vi "SVT UFF58 Write Record 8.vi"(0 "function refnum":refnum<k20>, 5 "abscissa data characteristics":T1 {"specific data type" items=["unknown"=0, "general"=1, "stress"=2, "strain"=3, "temperature"=5, "heat flux"=6, "displacement"=8, "reaction force"=9, "velocity"=11, "acceleration"=12, "excitation force"=13, "pressure"=15, "mass"=16, "time"=17, "frequency"=18, "rpm"=19, "order"=20, "sound pressure"=21, "sound intensity"=22, "sound power"=23]}, 11 "error in (no error)":errorcluster) -> (4 "dup function refnum":refnum<k20>, 15 "error out":errorcluster)   [LabVIEW 2017, in "SoundVib_UFF58.lvlib"]
doc: "Writes the values of the fields in record 8 of the UFF58 (universal file format) file. Record 8 contains the abscissa data characteristics."
uses:
  <vilib>/addons/Sound and Vibration/svt_UFF58/SoundVib_UFF58.lvlib
  <vilib>/addons/Sound and Vibration/svt_UFF58/subVIs/sv_UFF58 Axis Characteristics.ctl
  <vilib>/addons/Sound and Vibration/svt_UFF58/subVIs/sv_UFF58 Specific Datatype.ctl
  <vilib>/Platform/storage/Storage.llb/Set Property (String).vi
  <vilib>/Platform/storage/Storage.llb/Set Property (I32).vi
  <vilib>/Platform/storage/Storage.llb/Get Property (Storage Refnums).vi
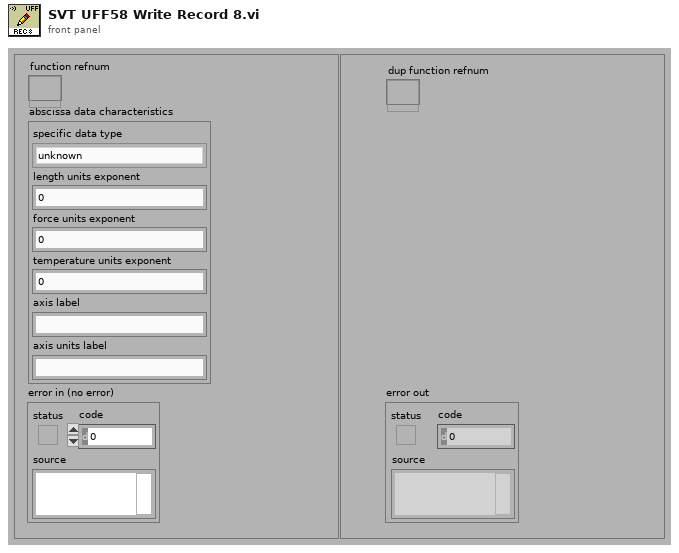
[diagram p1: front panel]
types:
  T1 = typedef "SoundVib_UFF58.lvlib/sv_UFF58 Axis Characteristics.ctl" = cluster{"specific data type":T2, "length units exponent":i32, "force units exponent":i32, "temperature units exponent":i32, "axis label":string, "axis units label":string}
  T2 = typedef "SoundVib_UFF58.lvlib/sv_UFF58 Specific Datatype.ctl" = u16
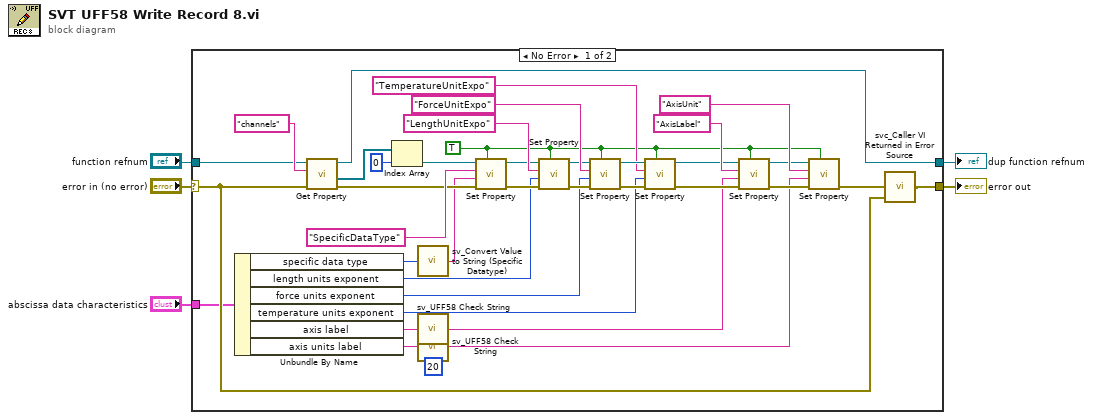
[diagram p0: block diagram]
diagram:
  n1 = case shown="No Error" "error in (no error)" {
    selector: "error in (no error)" -> [w10 w44]
    tunnel: [w12 w44] -> w5
    tunnel: "abscissa data characteristics" -> [w9 _]
    tunnel: "function refnum" -> [w17 w45]
    tunnel: [w14 w45] -> w1
    frame No Error {
      w8 = TRUE ("Create if not found (no:F)")
      w13 = 20 ("length (rest)")
      n2 = Unbundle By Name(w9) -> ("specific data type"=w6:T2, "length units exponent"=w25:i32, "force units exponent"=w24:i32, "temperature units exponent"=w23:i32, "axis label"=w27:string, "axis units label"=w26:string)
      n3 = call-poly <vilib>:"Get Property.vi"("error in (no error)"=w10, "Property name"="channels", "storage refnum"=w17) -> ("error out"=w16:errorcluster, "Value"=w19:refnum<k20>[], "storage refnum out"=w14:refnum<k20>)  [unwired: 6 in]
      n4 = Index Array(array=w19, index=0) -> (element=w15:refnum<k20>)
      n5 = call <vilib>:"sv_Convert Value to String (Specific Datatype).vi"("specific data type value"=w6) -> ("specific data type string"=w7:string)  [unwired: 14 in]
      n6 = call <vilib>:"sv_UFF58 Check String.vi"("field value"=w27, "field length"=w13) -> ("output string"=w21:string)  [unwired: 12 in, 1 out]
      n7 = call <vilib>:"sv_UFF58 Check String.vi"("field value"=w26, "field length"=w13) -> ("output string"=w22:string)  [unwired: 12 in, 1 out]
      n8 = call-poly <vilib>:"Set Property.vi"("Create if not found (no:F)"=w8, "error in (no error)"=w16, "Value"=w7, "Property name"="SpecificDataType", "storage refnum"=w15) -> ("error out"=w40:errorcluster, "storage refnum out"=w39:refnum<k20>)  [unwired: 5 in]
      n9 = call-poly <vilib>:"Set Property.vi"("Create if not found (no:F)"=w8, "error in (no error)"=w40, "Value"=w25, "Property name"="LengthUnitExpo", "storage refnum"=w39) -> ("error out"=w36:errorcluster, "storage refnum out"=w37:refnum<k20>)  [unwired: 5 in]
      n10 = call-poly <vilib>:"Set Property.vi"("Create if not found (no:F)"=w8, "error in (no error)"=w36, "Value"=w24, "Property name"="ForceUnitExpo", "storage refnum"=w37) -> ("error out"=w34:errorcluster, "storage refnum out"=w35:refnum<k20>)  [unwired: 5 in]
      n11 = call-poly <vilib>:"Set Property.vi"("Create if not found (no:F)"=w8, "error in (no error)"=w34, "Value"=w23, "Property name"="TemperatureUnitExpo", "storage refnum"=w35) -> ("error out"=w30:errorcluster, "storage refnum out"=w31:refnum<k20>)  [unwired: 5 in]
      n12 = call-poly <vilib>:"Set Property.vi"("Create if not found (no:F)"=w8, "error in (no error)"=w30, "Value"=w21, "Property name"="AxisLabel", "storage refnum"=w31) -> ("error out"=w28:errorcluster, "storage refnum out"=w29:refnum<k20>)  [unwired: 5 in]
      n13 = call-poly <vilib>:"Set Property.vi"("Create if not found (no:F)"=w8, "error in (no error)"=w28, "Value"=w22, "Property name"="AxisUnit", "storage refnum"=w29) -> ("error out"=w11:errorcluster)  [unwired: 5 in, 1 out]
      n14 = call <vilib>:"svc_Caller VI Returned in Error Source.vi"("warning input to caller"=w10, "error in (no error)"=w11) -> ("error out"=w12:errorcluster)  [unwired: 3 in]
    }
    frame Error {
    }
  }
  "error out" <- w5
  "dup function refnum" <- w1
